vi "Stopwatch Calc.vi"(8 "Reset":bool, 9 "Pause":bool, 10 "Play":bool, 11 "Stopwatch Data in":T1) -> (3 "Stopwatch Data out":T1)   [LabVIEW 2018]
uses:
  Shared Controls/Stopwatch Data.ctl
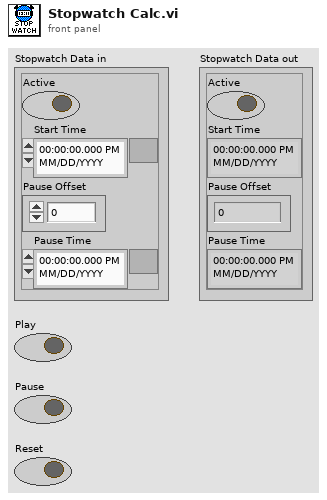
[diagram p1: front panel]
types:
  T1 = typedef "Stopwatch Data.ctl" = cluster{"Active":bool, "Start Time":timestamp, "Pause Offset":dbl, "Pause Time":timestamp}
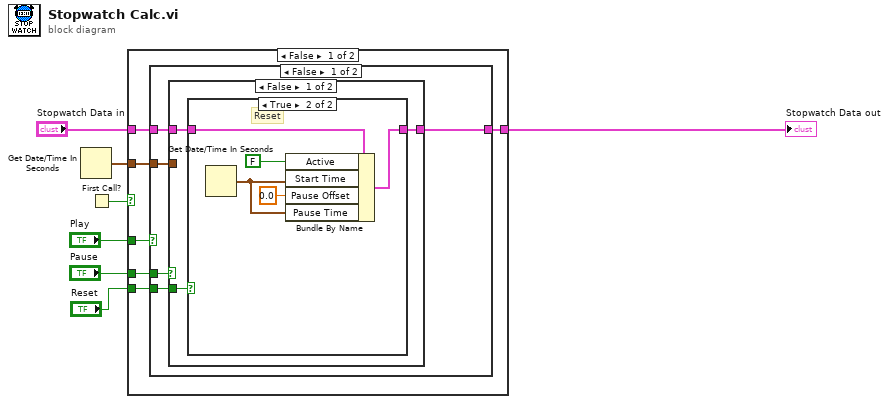
[diagram p0: block diagram]
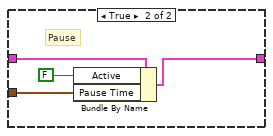
[diagram p3: hidden frame]
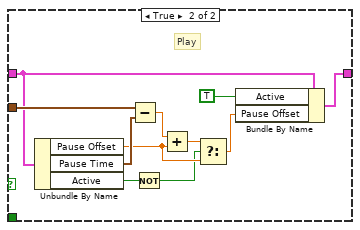
[diagram p4: hidden frame]
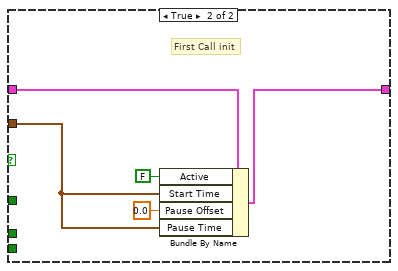
[diagram p5: hidden frame]
diagram:
  n1 = Get Date/Time In Seconds() -> (seconds since 1Jan1904=w5:timestamp)
  n2 = First Call?() -> (First Call?: T/F=w4:bool)
  n3 = case shown="False" w4 {
    tunnel: "Play" -> [w13 _]
    tunnel: "Pause" -> [w12 _]
    tunnel: "Reset" -> [w11 _]
    tunnel: w5 -> [w10 w44]
    tunnel: [w8 w45] -> w7
    tunnel: "Stopwatch Data in" -> [w9 w43]
    frame False {
      n4 = case shown="False" w13 {
        tunnel: w12 -> [w18 _]
        tunnel: w11 -> [w17 _]
        tunnel: w10 -> [w14 w35]
        tunnel: w9 -> [w15 w34]
        tunnel: [w16 w33] -> w8
        frame False {
          n5 = case shown="False" w18 {
            tunnel: w17 -> [w21 _]
            tunnel: [w20 w28] -> w16
            tunnel: w15 -> [w19 w29]
            tunnel: w14 -> [_ w30]
            frame False {
              n6 = case shown="True" w21 {
                tunnel: [w22 w23] -> w20
                tunnel: w19 -> [w22 w24]
                frame False {
                }
                frame True {
                  # "Reset"
                  n7 = Get Date/Time In Seconds() -> (seconds since 1Jan1904=w27:timestamp)
                  n8 = Bundle By Name(cluster=w24, "Active"=FALSE, "Start Time"=w27, "Pause Offset"=0.0, "Pause Time"=w27) -> (w23:T1)
                }
              }
            }
            frame True {
              # "Pause"
              n9 = Bundle By Name(cluster=w29, "Active"=FALSE, "Pause Time"=w30) -> (w28:T1)
            }
          }
        }
        frame True {
          # "Play"
          n10 = Unbundle By Name(w34) -> ("Pause Offset"=w40:dbl, "Pause Time"=w42:timestamp, "Active"=w37:bool)
          n11 = Subtract(x=w35, y=w42) -> (x-y=w39:dbl)
          n12 = Not(x=w37) -> (.not. x?=w32:bool)
          n13 = Add(x=w39, y=w40) -> (x+y=w38:dbl)
          n14 = Select(t=w38, s=w32, f=w40) -> (s? t:f=w41:dbl)
          n15 = Bundle By Name(cluster=w34, "Active"=TRUE, "Pause Offset"=w41) -> (w33:T1)
        }
      }
    }
    frame True {
      # "First Call init"
      n16 = Bundle By Name(cluster=w43, "Active"=FALSE, "Start Time"=w44, "Pause Offset"=0.0, "Pause Time"=w44) -> (w45:T1)
    }
  }
  "Stopwatch Data out" <- w7
